vi "Write then Read.vi"(8 "error in":errorcluster, 10 "write buffer":string, 11 "VISA resource name in":refnum<visa-resource-name>) -> (0 "error out":errorcluster, 2 "read buffer":string, 3 "VISA resource name out":refnum<visa-resource-name>)   [LabVIEW 2018, in "Support Library.lvlib"]
uses:
  Support Library.lvlib
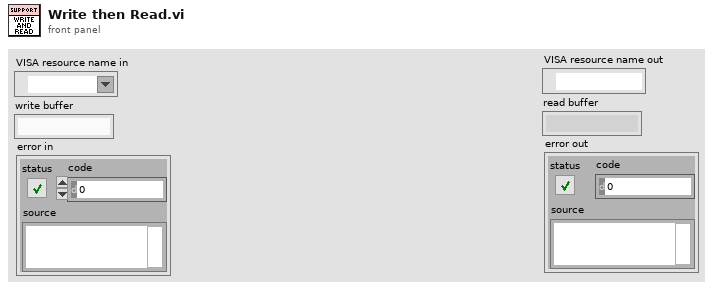
[diagram p1: front panel]
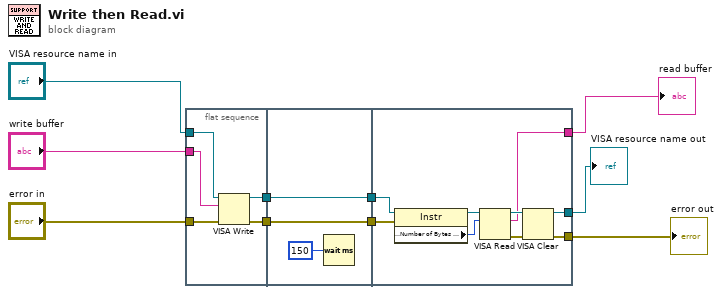
[diagram p0: block diagram]
diagram:
  n1 = flat-sequence {
    tunnel: [w14] -> w10
    tunnel: [w15] -> w9
    tunnel: "write buffer" -> [w13]
    tunnel: "VISA resource name in" -> [w12]
    tunnel: "error in" -> [w11]
    tunnel: w10 -> [w18]
    tunnel: w9 -> [w17]
    tunnel: [w18] -> w8
    tunnel: [w17] -> w7
    tunnel: [w21] -> w6
    tunnel: [w23] -> w4
    tunnel: w8 -> [w22]
    tunnel: w7 -> [w24]
    tunnel: [w20] -> w5
    frame #0 {
      n2 = VISA Write(VISA resource name=w12, write buffer=w13, error in (no error)=w11) -> (VISA resource name out=w15:refnum<visa-resource-name>, error out=w14:errorcluster)  [unwired: 1 out]
    }
    frame #1 {
      n3 = Wait (ms)(milliseconds to wait=u32 150) -> ()  [unwired: 1 out]
    }
    frame #2 {
      n4 = property class="Instr"(reference=w24, error in=w22) -> (reference out=w27:refnum<visa-resource-name>, "Serial Settings:Number of Bytes at Serial Port"=w19:u32)  [unwired: 1 out]
      n5 = VISA Read(VISA resource name=w27, byte count=w19) -> (VISA resource name out=w25:refnum<visa-resource-name>, read buffer=w20:string, error out=w26:errorcluster)  [unwired: 1 in, 1 out]
      n6 = VISA Clear(VISA resource name=w25, error in (no error)=w26) -> (VISA resource name out=w21:refnum<visa-resource-name>, error out=w23:errorcluster)
    }
  }
  "VISA resource name out" <- w6
  "read buffer" <- w5
  "error out" <- w4
